vi "Time Formatting.vi"(0 "NMEA Input":string) -> (1 "GPS UTC":timestamp, 2 "UNIX Timestamp":u32)   [LabVIEW 2016]
panel:
  # "This converts the GPS NMEA sentence into time and date formats"
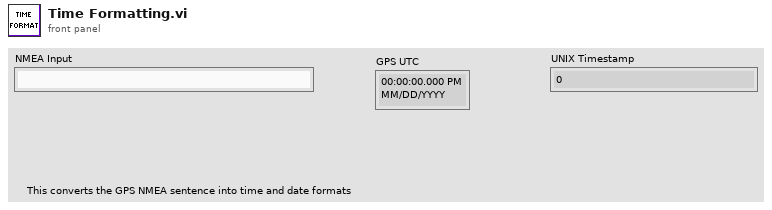
[diagram p1: front panel]
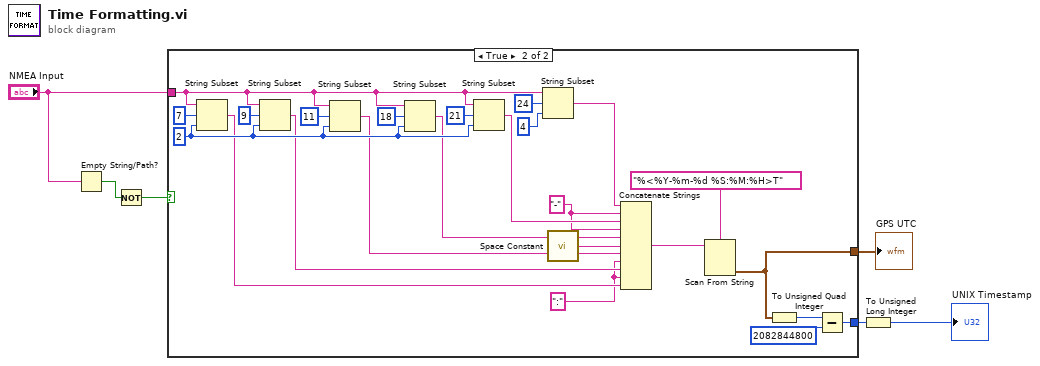
[diagram p0: block diagram]
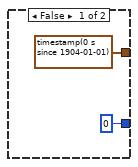
[diagram p2: hidden frame]
diagram:
  n1 = Empty String/Path?(string/path="NMEA Input") -> (empty?=w3:bool)
  n2 = Not(x=w3) -> (.not. x?=w4:bool)
  n3 = case shown="True" w4 {
    tunnel: "NMEA Input" -> [_ w28]
    tunnel: [timestamp(0 s since 1904-01-01) w12] -> w6
    tunnel: [u64 0 w9] -> w2
    frame False {
    }
    frame True {
      w15 = ":"
      w17 = "-"
      w25 = 2 ("length (rest)")
      n4 = String Subset(string=w28, offset (0)=7, length (rest)=w25) -> (substring=w18:string)
      n5 = String Subset(string=w28, offset (0)=9, length (rest)=w25) -> (substring=w19:string)
      n6 = String Subset(string=w28, offset (0)=11, length (rest)=w25) -> (substring=w20:string)
      n7 = String Subset(string=w28, offset (0)=18, length (rest)=w25) -> (substring=w21:string)
      n8 = String Subset(string=w28, offset (0)=21, length (rest)=w25) -> (substring=w22:string)
      n9 = String Subset(string=w28, offset (0)=24, length (rest)=4 ("length (rest)")) -> (substring=w23:string)
      n10 = call <vilib>:"Space Constant.vi"() -> ("String"=w16:string)
      n11 = Concatenate Strings(w23, w17, w22, w17, w21, w16, w20, w15, w19, w15, w18) -> (w13:string)
      n12 = Scan From String(format string="%<%Y-%m-%d %S:%M:%H>T", input string=w13) -> (output 1=w12:timestamp)  [unwired: 3 in, 3 out]
      n13 = To Unsigned Quad Integer(1:w12) -> (0:w11:u64)
      n14 = Subtract(x=w11, y=u64 2082844800) -> (x-y=w9:u64)
    }
  }
  "GPS UTC" <- w6
  n15 = To Unsigned Long Integer(number=w2) -> (unsigned 32bit integer=→"UNIX Timestamp":u32)
